vi "Get Enable State.vi"(8 "error in (no error)":errorcluster, 11 "hdl":i32) -> (0 "error out":errorcluster, 2 "Enable":bool, 3 "hdl out":i32)   [LabVIEW 2018, in "Thorlabs_SC10.lvlib"]
uses:
  Thorlabs_SC10.lvlib
  SC10CommandLib_x64.dll
  SC10CommandLib_win32.dll
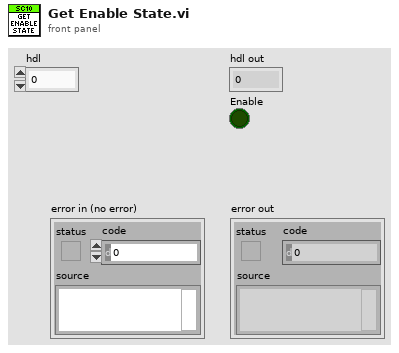
[diagram p1: front panel]
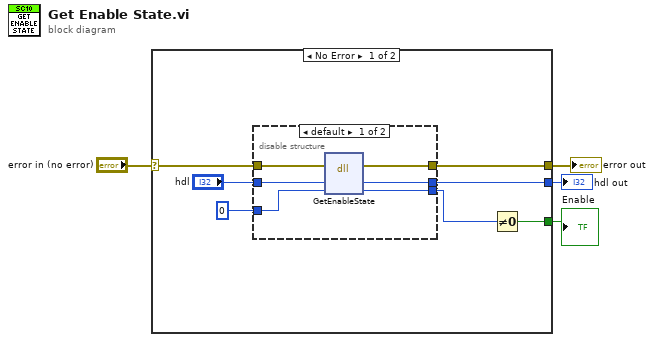
[diagram p0: block diagram]
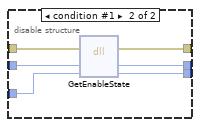
[diagram p2: hidden frame]
diagram:
  n1 = case shown="No Error" "error in (no error)" {
    selector: "error in (no error)" -> [w11 w24]
    tunnel: [w7 w24] -> w4
    tunnel: [w10 _] -> w2
    tunnel: [w5 _] -> w1
    frame No Error {
      n2 = disable-structure shown="default" {
        disable-tunnel: w11 -> [w17 w23]
        disable-tunnel: [w16 w22] -> w7
        disable-tunnel: [w15 w21] -> w10
        disable-tunnel: "hdl" -> [w14 w20]
        disable-tunnel: 0 ("value") -> [w13 w19]
        disable-tunnel: [w12 w18] -> w6
        frame condition #0 (active) {
          n3 = dll-call lib="C:/Program Files (x86)/National Instruments/LabVIEW 2018/instr.lib/Thorlabs_SC10/Data/SC10CommandLib_win32.dll" fn="GetEnableState"(error in=w17, "hdl"=w14, "value"=w13) -> (error out=w16:errorcluster, "hdl"=w15:i32, "value"=w12:i32)  [unwired: 3 in, 1 out]
        }
        frame condition #1 {
          n4 = dll-call lib="C:/Program Files/National Instruments/LabVIEW 2011/instr.lib/Thorlabs_SC10/Data/SC10CommandLib_x64.dll" fn="GetEnableState"(error in=w23, "hdl"=w20, "value"=w19) -> (error out=w22:errorcluster, "hdl"=w21:i32, "value"=w18:i32)  [unwired: 3 in, 1 out]
        }
      }
      n5 = Not Equal To 0?(x=w6) -> (x != 0?=w5:bool)
    }
    frame Error {
    }
  }
  "error out" <- w4
  "hdl out" <- w2
  "Enable" <- w1
